vi "CoherenceTest.vi"() -> ()   [LabVIEW 2017]
uses:
  <vilib>/Platform/TimedLoop/XDataNode/timing_clust.ctl
  <vilib>/Platform/TimedLoop/XDataNode/nitl_modes.ctl
  <vilib>/Platform/TimedLoop/XDataNode/wakeup.ctl
  <vilib>/Analysis/baseanly.llb/Normalize Vector.vi
  <vilib>/Analysis/baseanly.llb/Quick Scale 1D.vi
  <vilib>/DAQmx/write.llb/DAQmx Write (Analog 2D DBL NChan NSamp).vi
  <vilib>/DAQmx/create/channels.llb/DAQmx Create Channel (AO-Voltage-Basic).vi
  <vilib>/DAQmx/configure/timing.llb/DAQmx Timing (Sample Clock).vi
  <vilib>/Analysis/3filter.llb/IIR Filter (DBL).vi
  <vilib>/DAQmx/miscellaneous.llb/DAQmx Fill In Error Info.vi
  <vilib>/platform/TimedLoop/XDataNode/XDataNode.xnode
  <vilib>/Analysis/NI_AALBase.lvlib
  <vilib>/Platform/TimedLoop/XDataNode/XDNodeRunTimeDep.lvlib
panel:
  out "Coherence plot":dbl[](graph)
  out "Coherence at sinusoid frequency":dbl format="%#_4g"
  in  "SNR":dbl=1.0 min=0.0
  in  "Sinusoid frequency":dbl=10.0
  out "Error":errorcluster
  in  "Max amplitude":dbl=1.0 format="%0.2f"
  in  "Output terminals":tag="PCI-DAQ/ao0:1"
  in  "stop":bool
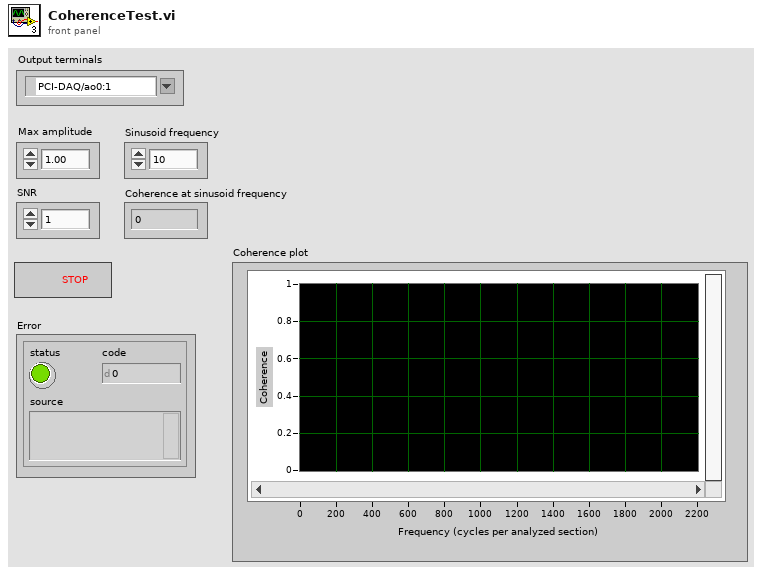
[diagram p1: front panel]
types:
  T1 = typedef "XDNodeRunTimeDep.lvlib/timing_clust.ctl" = cluster{"Expected End [f-1]":u64, "Actual End [f-1]":u64, "Finished Late? [f-1]":bool, "Expected End [i-1]":u64, "Actual End [i-1]":u64, "Finished Late? [i-1]":bool, "Expected Start [i]":u64, "Actual Start [i]":u64, "Expected Start [f]":u64, "Actual Start [f]":u64, "Source Name":string, "Structure Name":string, "Period":i64, "Deadline":i64, "Offset":i64, "Start":i64, "Priority":i32, "Timeout":i32, "Mode":T2, "Wakeup Reason":T3, "Error":errorcluster, "Source Type":string, "Secondary Source Type":string, "Global End Time":u64, "Global Start Time":u64, "Frame Duration":u64, "Iteration Duration":u64, "Assigned CPU":i32, "I/O Scan Engine Mode":u32}
  T2 = typedef "XDNodeRunTimeDep.lvlib/nitl_modes.ctl" = enum32{"No Change", "Process missed periods, maintain original phase", "Discard missed periods, maintain original phase", "Process missed periods, ignore original phase", "Discard missed periods, ignore original phase"}
  T3 = typedef "XDNodeRunTimeDep.lvlib/wakeup.ctl" = enum32{"Normal", "Aborted", "Asynchronous wakeup", "Timing source error", "Timed loop error", "Timeout"}
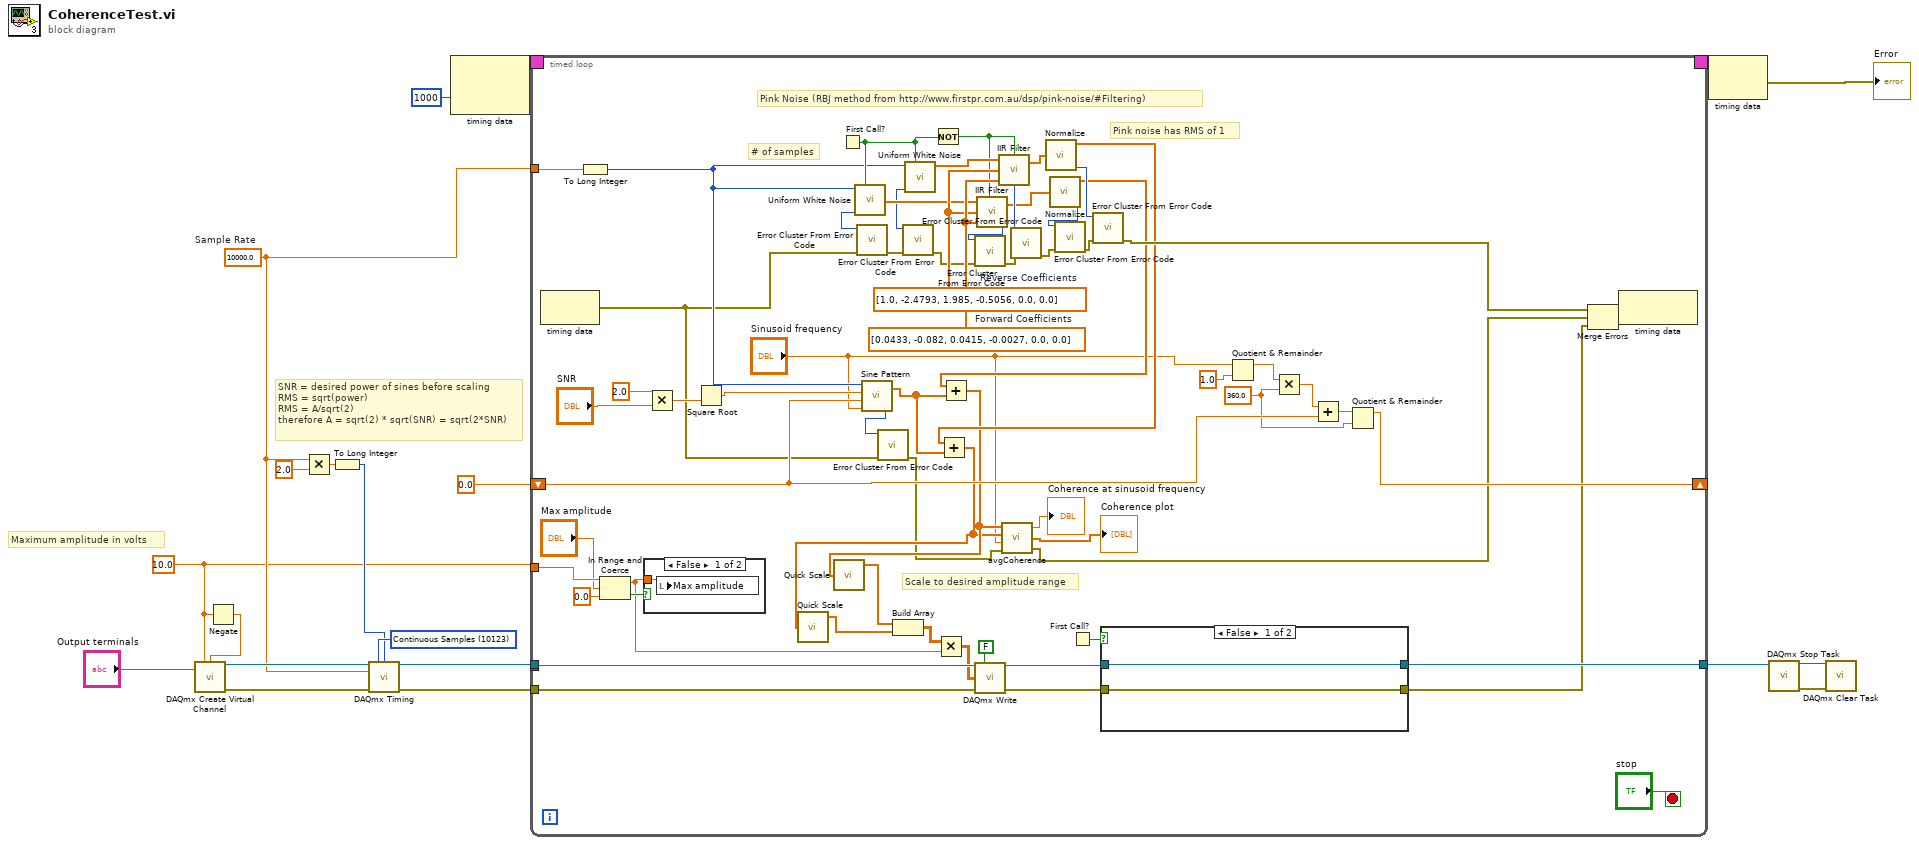
[diagram p0: block diagram]
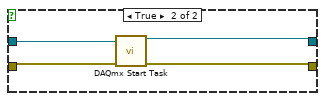
[diagram p3: hidden frame]
diagram:
  w4 = 10.0 ("x")
  w9 = 10000.0  # Sample Rate
  w10 = 10123 items=["Finite Samples"=10178, "Continuous Samples"=10123, "Hardware Timed Single Point"=12522] ("sample mode")
  # "SNR = desired power of sines before scaling\nRMS = sqrt(power)\nRMS = A/sqrt(2)\ntherefore A = sqrt(2) * sqrt(SNR) = sqrt(2*SNR)"
  # "Maximum amplitude in volts"
  n1 = Negate(x=w4) -> (-x=w3:dbl)
  n2 = call-poly <vilib>:"DAQmx Create Virtual Channel.vi"("maximum value"=w4, "minimum value"=w3, "physical channels"="Output terminals") -> ("task out"=w14:refnum<k21>, "error out"=w13:errorcluster)  [unwired: 11 in]
  n3 = Multiply(x=w9, y=2.0) -> (x*y=w7:dbl)
  n4 = To Long Integer(number=w7) -> (32bit integer=w6:i32)
  n5 = call-poly <vilib>:"DAQmx Timing.vi"("task/channels in"=w14, "sample mode"=w10, "samples per channel"=w6, "rate"=w9, "error in"=w13) -> ("task out"=w11:refnum<k21>, "error out"=w12:errorcluster)  [unwired: 9 in]
  n6 = node-c288(i64 1000 ("Period")) -> (w20:T1)  [unwired: 1 in]
  n7 = timed-loop {
    timing: w20 -> [_]
    timing-out: [_] -> w19
    tunnel: [w66] -> _
    tunnel: w11 -> [w66]
    tunnel: w12 -> [w80]
    tunnel: [w79] -> w17
    tunnel: w9 -> [w46]
    tunnel: w4 -> [w55]
    shift-right: [w38] -> _
    shift-left: 0.0 -> [w41]
    stop <- "stop" stop-if-true
    w40 = 360.0 ("y")
    w77 = dbl[] [0.0433, -0.082, 0.0415, -0.0027, 0.0, 0.0]  # Forward Coefficients
    w76 = dbl[] [1.0, -2.4793, 1.985, -0.5056, 0.0, 0.0]  # Reverse Coefficients
    # "Pink noise has RMS of 1"
    # "Scale to desired amplitude range"
    # "# of samples"
    # "Pink Noise (RBJ method from http://www.firstpr.com.au/dsp/pink-noise/#Filtering)"
    n8 = node-c288() -> (w26:errorcluster)  [unwired: 1 in]
    n9 = To Long Integer(number=w46) -> (32bit integer=w45:i32)
    n10 = In Range and Coerce(upper limit=w55, x="Max amplitude", lower limit=0.0) -> (coerced(x)=w52:dbl, In Range?=w53:bool)
    n11 = case shown="False" w53 {
      tunnel: w52 -> [w84 _]
      frame False {
        n12 = local write "Max amplitude"(w84) -> ()
      }
      frame True {
      }
    }
    n13 = Multiply(x=2.0, y="SNR") -> (x*y=w35:dbl)
    n14 = Square Root(x=w35) -> (sqrt(x)=w34:dbl)
    n15 = First Call?() -> (First Call?: T/F=w78:bool)
    n16 = call <vilib>:"Uniform White Noise.vi"("initialize?"=w78, "samples"=w45) -> ("error"=w71:i32, "uniform white noise"=w75:dbl[])  [unwired: 8 in]
    n17 = call <vilib>:"Error Cluster From Error Code.vi"("error in (no error)"=w26, "error code (0)"=w71) -> ("error out"=w70:errorcluster)  [unwired: 7 in]
    n18 = call <vilib>:"Sine Pattern.vi"("cycles"="Sinusoid frequency", "phase(degrees)"=w41, "amplitude"=w34, "samples"=w45) -> ("error"=w27:i32, "Sinusoidal Pattern"=w31:dbl[])
    n19 = call <vilib>:"Error Cluster From Error Code.vi"("error in (no error)"=w26, "error code (0)"=w27) -> ("error out"=w25:errorcluster)  [unwired: 7 in]
    n20 = call <vilib>:"Uniform White Noise.vi"("initialize?"=w78, "samples"=w45) -> ("error"=w72:i32, "uniform white noise"=w82:dbl[])  [unwired: 8 in]
    n21 = call <vilib>:"Error Cluster From Error Code.vi"("error in (no error)"=w70, "error code (0)"=w72) -> ("error out"=w69:errorcluster)  [unwired: 7 in]
    n22 = Not(x=w78) -> (.not. x?=w74:bool)
    n23 = call-poly <vilib>:"IIR Filter.vi"("init/cont (init:F)"=w74, "Forward Coefficients"=w77, "Reverse Coefficients"=w76, "X"=w75) -> ("error"=w68:i32, "Filtered X"=w62:dbl[])
    n24 = call <vilib>:"Error Cluster From Error Code.vi"("error in (no error)"=w69, "error code (0)"=w68) -> ("error out"=w67:errorcluster)  [unwired: 7 in]
    n25 = call-poly <vilib>:"IIR Filter.vi"("init/cont (init:F)"=w74, "Forward Coefficients"=w77, "Reverse Coefficients"=w76, "X"=w82) -> ("error"=w73:i32, "Filtered X"=w63:dbl[])
    n26 = call <vilib>:"Error Cluster From Error Code.vi"("error in (no error)"=w67, "error code (0)"=w73) -> ("error out"=w59:errorcluster)  [unwired: 7 in]
    n27 = call-poly <vilib>:"Normalize.vi"("Vector"=w63) -> ("error"=w49:i32, "Normalized Vector"=w32:dbl[])  [unwired: 1 in, 2 out]
    n28 = Add(x=w32, y=w31) -> (x+y=w29:dbl[])
    n29 = call-poly <vilib>:"Quick Scale.vi"("X"=w29) -> ("Y[i]=X[i]/Max|X|"=w47:dbl[])  [unwired: 2 out]
    n30 = call-poly <vilib>:"Normalize.vi"("Vector"=w62) -> ("error"=w51:i32, "Normalized Vector"=w33:dbl[])  [unwired: 1 in, 2 out]
    n31 = Add(x=w33, y=w31) -> (x+y=w30:dbl[])
    n32 = call-poly <vilib>:"Quick Scale.vi"("X"=w30) -> ("Y[i]=X[i]/Max|X|"=w48:dbl[])  [unwired: 2 out]
    n33 = Build Array(w48, w47) -> (w60:dbl[][])
    n34 = Multiply(x=w60, y=w52) -> (x*y=w61:dbl[][])
    n35 = call-poly <vilib>:"DAQmx Write.vi"("task/channels in"=w66, "auto start"=FALSE, "data"=w61) -> ("task out"=w65:refnum<k21>)  [unwired: 10 in, 2 out]
    n36 = call "avgCoherence.vi"("error in (no error)"=w25, "frequency (cycles/period)"="Sinusoid frequency", "x2"=w29, "x1"=w30) -> ("error out"=w24:errorcluster, "coherence"=→"Coherence plot":dbl[], "coherence at frequency"=→"Coherence at sinusoid frequency":dbl)
    n37 = call <vilib>:"Error Cluster From Error Code.vi"("error in (no error)"=w59, "error code (0)"=w51) -> ("error out"=w50:errorcluster)  [unwired: 7 in]
    n38 = First Call?() -> (First Call?: T/F=w81:bool)
    n39 = call <vilib>:"Error Cluster From Error Code.vi"("error in (no error)"=w50, "error code (0)"=w49) -> ("error out"=w57:errorcluster)  [unwired: 7 in]
    n40 = case shown="False" w81 {
      tunnel: w65 -> [w86 w87]
      tunnel: w80 -> [w85 w88]
      tunnel: [w85 w89] -> w23
      tunnel: [w86 w90] -> w79
      frame False {
      }
      frame True {
        n41 = call <vilib>:"DAQmx Start Task.vi"("task/channels in"=w87, "error in"=w88) -> ("task out"=w90:refnum<k21>, "error out"=w89:errorcluster)  [unwired: 12 in]
      }
    }
    n42 = Quotient & Remainder(x="Sinusoid frequency", y=1.0) -> (x-y*floor(x/y)=w39:dbl)  [unwired: 1 out]
    n43 = Multiply(x=w39, y=w40) -> (x*y=w43:dbl)
    n44 = Add(x=w43, y=w41) -> (x+y=w42:dbl)
    n45 = Quotient & Remainder(x=w42, y=w40) -> (x-y*floor(x/y)=w38:dbl)  [unwired: 1 out]
    n46 = Merge Errors(w57, w24, w23) -> (w58:errorcluster)
    n47 = node-c288(w58) -> ()  [unwired: 1 out]
  }
  n48 = node-c288(w19) -> (→"Error":errorcluster)
  n49 = call <vilib>:"DAQmx Stop Task.vi"("task/channels in"=w17) -> ("task out"=w16:refnum<k21>, "error out"=w15:errorcluster)  [unwired: 13 in]
  n50 = call <vilib>:"DAQmx Clear Task.vi"("task in"=w16, "error in"=w15) -> ()  [unwired: 13 in, 1 out]
